vi "Record Players.vi"(10 "Password":string, 11 "Internal Data In":T1) -> (1 "resume?":bool, 2 "verified?":bool, 3 "Internal Data Out":T1)   [LabVIEW 2025]
uses:
  Internal Data.ctl
  Collision Box.ctl
  <vilib>/picture/picture.llb/imagedata.ctl
  <vilib>/Utility/config.llb/Read Key (String).vi
  <vilib>/Utility/config.llb/Read Key (I32).vi
  <vilib>/Utility/config.llb/Write Key (String).vi
  <vilib>/Utility/config.llb/Write Key (I32).vi
  <vilib>/Utility/config.llb/NI_LVConfig.lvlib
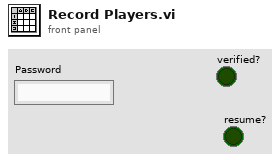
[diagram p1: front panel]
types:
  T1 = typedef "Internal Data.ctl" = cluster{"Core":cluster{"Current VI Reference":refnum<vi>, "Close Panel on Exit?":bool}, "Collision Box":T2, "Walls":cluster{"[0]":T3, "[1]":T3, "[2]":T3, "[3]":T3, "[4]":T3, "[5]":T3, "[6]":T3, "[7]":T3, "[8]":T3}, "Floor":T3, "Gates":cluster{"[0]":T3, "[1]":T3, "[2]":T3, "[3]":T3, "[4]":T3, "[5]":T3, "[6]":T3, "[7]":T3, "[8]":T3}, "Gate Condition":bool[], "Level":i32, "Score":i32, "Player Image":T3, "Display Font":cluster{"Font Name:":string, "Size":i16, "Strikeout?":bool, "Italic?":bool, "Underline?":bool, "Outline?":bool, "Shadow?":bool, "Bold?":bool}, "Menu Image":T3, "Menu Button Image":T3, "Menu Selected Image":T3, "Menu Selection":i32, "Player Name":string, "Menu Wall Image":T3}
  T2 = typedef "Collision Box.ctl" = cluster{"left":i16, "top":i16, "right":i16, "bottom":i16}
  T3 = typedef "imagedata.ctl" = cluster{"image type":i32, "image depth":i32, "image":u8[], "mask":u8[], "colors":u32[], "Rectangle":cluster{"left":i16, "top":i16, "right":i16, "bottom":i16}}
  T4 = typedef "NI_LVConfig.lvlib/Config Data RefNum.ctl" = refnum<k1>
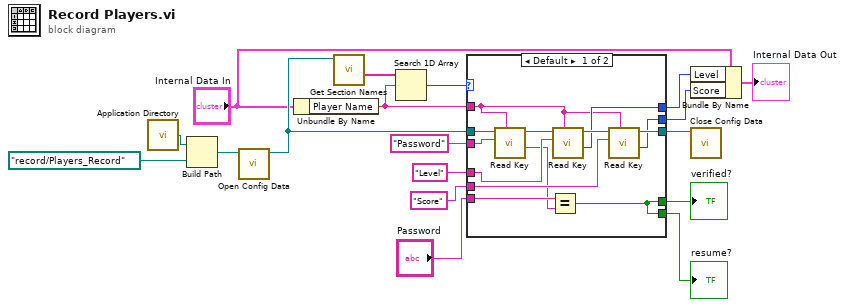
[diagram p0: block diagram]
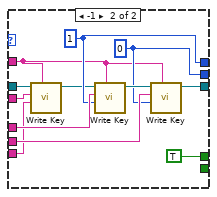
[diagram p2: hidden frame]
diagram:
  n1 = call <vilib>:"Application Directory.vi"() -> ("Application Directory"=w18:path)
  n2 = Build Path(base path=w18, name or relative path=path "record/Players_Record") -> (appended path=w16:path)
  n3 = call <vilib>:"Open Config Data.vi"("configuration file path"=w16) -> ("refnum"=w12:T4)  [unwired: 8 in, 2 out]
  n4 = Unbundle By Name("Internal Data In") -> ("Player Name"=w13:string)
  n5 = call <vilib>:"Get Section Names.vi"("refnum"=w12) -> ("section names"=w15:string[])  [unwired: 8 in, 2 out]
  n6 = Search 1D Array(1D array=w15, element=w13) -> (index of element=w14:i32)  [unwired: 1 in]
  n7 = case shown="Default" w14 {
    tunnel: w13 -> [w23 w33]
    tunnel: w12 -> [w25 w37]
    tunnel: [w30 w42] -> w11
    tunnel: [w29 w38] -> w8
    tunnel: [w28 w39] -> w7
    tunnel: "Level" ("key") -> [w27 w41]
    tunnel: "Score" ("key") -> [w26 w40]
    tunnel: "Password" -> [w22 w35]
    tunnel: "Password" -> [w21 w34]
    tunnel: [w19 TRUE] -> w2
    tunnel: [w19 _] -> w1
    frame Default {
      n8 = call-poly <vilib>:"Read Key.vi"("section"=w23, "key"=w22, "refnum"=w25) -> ("value"=w20:string, "refnum out"=w24:T4)  [unwired: 5 in, 2 out]
      n9 = Equal?(x=w21, y=w20) -> (x = y?=w19:bool)
      n10 = call-poly <vilib>:"Read Key.vi"("section"=w23, "key"=w27, "refnum"=w24) -> ("value"=w29:i32, "refnum out"=w31:T4)  [unwired: 5 in, 2 out]
      n11 = call-poly <vilib>:"Read Key.vi"("section"=w23, "key"=w26, "refnum"=w31) -> ("value"=w28:i32, "refnum out"=w30:T4)  [unwired: 5 in, 2 out]
    }
    frame -1 {
      w38 = 1
      w39 = 0
      n12 = call-poly <vilib>:"Write Key.vi"("section"=w33, "value"=w34, "key"=w35, "refnum"=w37) -> ("refnum out"=w36:T4)  [unwired: 5 in, 2 out]
      n13 = call-poly <vilib>:"Write Key.vi"("section"=w33, "value"=w38, "key"=w41, "refnum"=w36) -> ("refnum out"=w43:T4)  [unwired: 5 in, 2 out]
      n14 = call-poly <vilib>:"Write Key.vi"("section"=w33, "value"=w39, "key"=w40, "refnum"=w43) -> ("refnum out"=w42:T4)  [unwired: 5 in, 2 out]
    }
  }
  "verified?" <- w2
  "resume?" <- w1
  n15 = Bundle By Name(cluster="Internal Data In", "Level"=w8, "Score"=w7) -> (→"Internal Data Out":T1)
  n16 = call <vilib>:"Close Config Data.vi"("refnum"=w11) -> ()  [unwired: 9 in, 2 out]
